vi "Write Library Path.vi"(8 "error in (no error)":errorcluster, 10 "Library Path":path, 11 "Library in":refnum<class "Library.lvclass">) -> (0 "error out":errorcluster, 3 "Library out":refnum<class "Library.lvclass">)   [LabVIEW 2019, in "Panther Dashboard.lvlib" / "Library.lvclass"]
uses:
  Library.lvclass
  Library.lvclass/Library.ctl
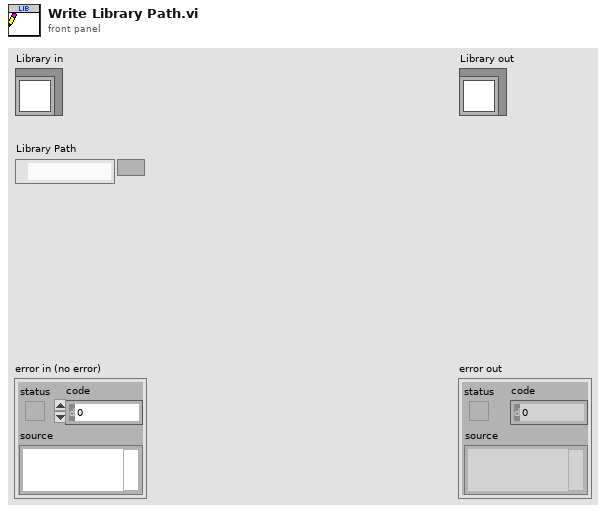
[diagram p1: front panel]
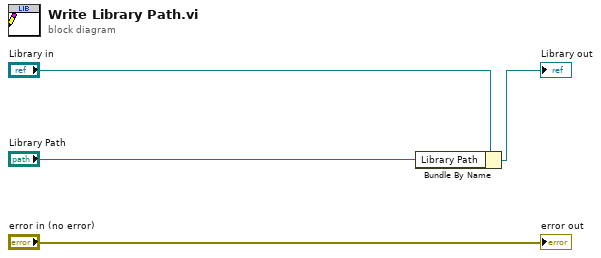
[diagram p0: block diagram]
diagram:
  n1 = Bundle By Name(cluster="Library in", "Library Path"="Library Path") -> (→"Library out":refnum<class "Library.lvclass">)
  "error out" <- "error in (no error)"
